vi "PXI - Route Trigger.vi"() -> ()   [LabVIEW 2023]
doc: "This example opens a session to a PXI BACKPLANE resource and routes trigger lines for an identified PXI system. The PXI BACKPLANE resource follows the format \n\nPXI0::?::BACKPLANE \n\nwhere ? is the number of the PXI chassis in NI MAX (Measurement & Automation Explorer). \n\n<b>Note:</b> This VI routes triggers from a source bus to a destination bus but does not reserve a trigger line in the source bus. This can allow multiple boards to drive a single trigger line, which can damage hardware. \n\nRefer to the PXI - Reserve Trigger.vi example for an example of reserving the source trigger so that automatic drivers, such as NI-DAQmx, do not use the same line."
panel:
  in  "Source Trigger Bus":i16=1
  in  "Destination Trigger Bus":i16=3
  in  "PXI Trigger Number":i16
  in  "Unroute Trigger":bool
  in  "Stop":bool
  in  "PXI Backplane VISA resource name":refnum<visa-resource-name>
  in  "Route Trigger":bool
  # "Overview: Demonstrates the use of the VISA functions to route a trigger on a PXI backplane.\nRequirements: NI-VISA Driver, PXI device\nInstructions:\n1. Ensure the device specified by the PXI Backplane VISA resource name control is properly configured in Measurement & Automation Explorer.\n2. Run the VI.\n3. Click the Route Trigger and Unroute Trigger buttons to manipulate the PXI backplane trigger.\n4. Click Stop to stop the VI."
  # "Note: This example does not reserve the source trigger line."
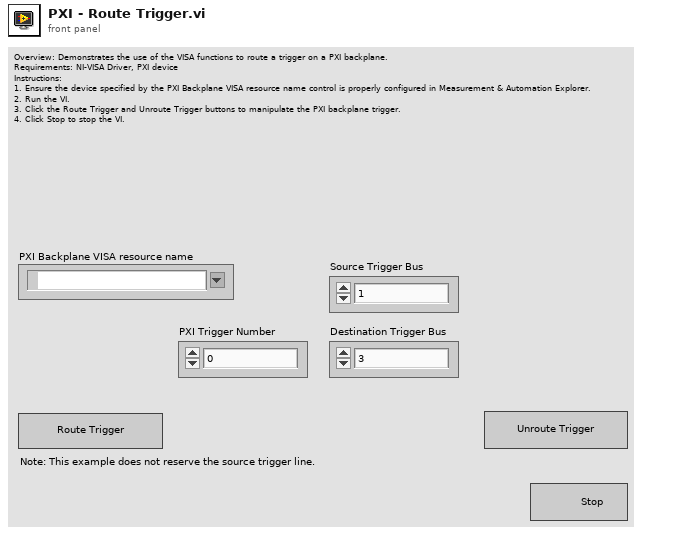
[diagram p1: front panel]
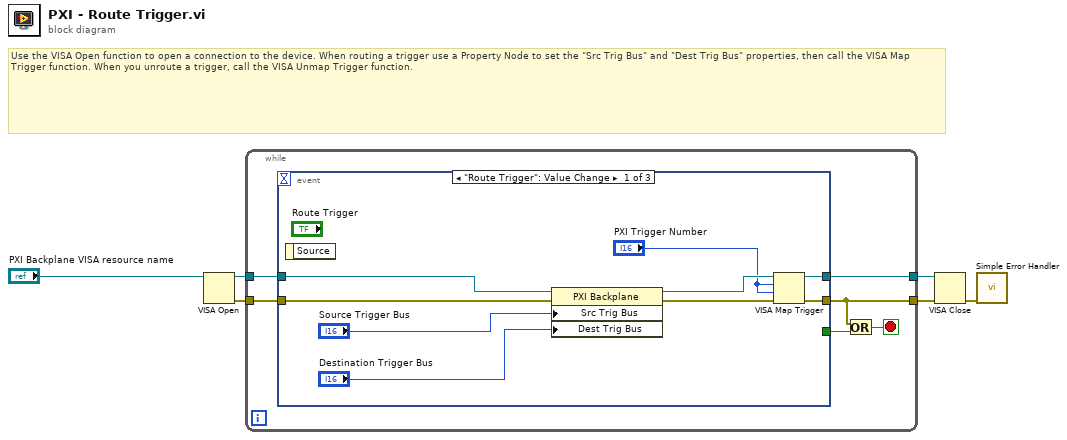
[diagram p0: block diagram]
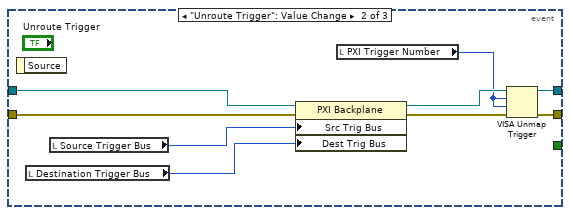
[diagram p2: hidden frame]
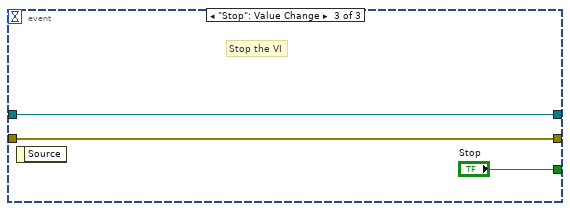
[diagram p3: hidden frame]
diagram:
  # "Use the VISA Open function to open a connection to the device. When routing a trigger use a Property Node to set the \"Src Trig Bus\" and \"Dest Trig Bus\" properties, then call the VISA Map Trigger function. When you unroute a trigger, call the VISA Unmap Trigger function."
  n1 = VISA Open(VISA resource name="PXI Backplane VISA resource name") -> (VISA resource name=w4:refnum<visa-resource-name>, error out=w5:errorcluster)  [unwired: 1 in, 3 out]
  n2 = while {
    tunnel: w4 -> [w9]
    tunnel: [w10] -> w1
    tunnel: w5 -> [w7]
    tunnel: [w8] -> w3
    stop <- w11 stop-if-true
    n3 = event shown="[0] \"Route Trigger\": Value Change" {
      selector: _ -> [_ _ _]
      dyn-events: _ -> [_ _ _]
      timeout: _ -> [_ _ _]
      tunnel: [_ _ "Stop"] -> w12
      tunnel: [w20 w29 w32] -> w8
      tunnel: w7 -> [w18 w25 w32]
      tunnel: [w21 w30 w31] -> w10
      tunnel: w9 -> [w19 w28 w31]
      event "Route Trigger": Value Change {
        n4 = event-data() -> ()  [unwired: 2 out]
        n5 = property class="PXI Backplane"(reference=w19, error in=w18, "Src Trig Bus"="Source Trigger Bus", "Dest Trig Bus"="Destination Trigger Bus") -> (reference out=w16:refnum<visa-resource-name>, error out=w17:errorcluster)
        n6 = VISA Map Trigger(8:w17, 9:"PXI Trigger Number", 10:"PXI Trigger Number", 11:w16) -> (0:w20:errorcluster, 3:w21:refnum<visa-resource-name>)  [unwired: 1 in]
      }
      event "Unroute Trigger": Value Change {
        n7 = event-data() -> ()  [unwired: 2 out]
        n8 = local read "Destination Trigger Bus"() -> (w22:i16)
        n9 = local read "Source Trigger Bus"() -> (w23:i16)
        n10 = property class="PXI Backplane"(reference=w28, error in=w25, "Src Trig Bus"=w23, "Dest Trig Bus"=w22) -> (reference out=w27:refnum<visa-resource-name>, error out=w26:errorcluster)
        n11 = local read "PXI Trigger Number"() -> (w24:i16)
        n12 = VISA Unmap Trigger(8:w26, 9:w24, 10:w24, 11:w27) -> (0:w29:errorcluster, 3:w30:refnum<visa-resource-name>)
      }
      event "Stop": Value Change {
        # "Stop the VI"
        n13 = event-data() -> ()  [unwired: 2 out]
      }
    }
    n14 = Or(x=w8, y=w12) -> (x .or. y?=w11:bool)
  }
  n15 = VISA Close(VISA resource name=w1, error in (no error)=w3) -> (error out=w2:errorcluster)
  n16 = call <vilib>:"Simple Error Handler.vi"("error in (no error)"=w2) -> ()  [unwired: 1 in, 8 out]
